vi "write_test_section_data.vi"(0 "dequeued data":T1={"Vapor Flow rate [g/s]"=0.0, "Liquid Flow rate [g/s]"=0.0, "Pressure/Temperature/Mixture Properties"={"Line Densities\n[g/cm^3]"={"Vapor Line"=0.15445189986836314, "Liquid Line"=0.25755261741892205}, "Mixture Properties"={"Enthalpy"=195841526251804.2, "Quality [-]"=-10.825375459319764}, "[Readings]"={"Streamwise P"=-3074.4228785963764, "Streamwise T"=nan, "Streamwise Sat P"=nan, "Streamwise Sat T"=nan, "Liquid Tank P"=3834985507386.06, "Liquid Tank T"=456.4106234658312, "Liquid Tank Sat P"=1736233577203.0627, "Liquid Tank Sat T"=492.17973224367375, "Separator P"=179910.46497250997, "Separator T"=-13120080.345725078, "Separator Sat P"=0.0, "Separator Sat T"=30.62899308837065, "Liquid Inlet P"=185261.09355383943, "Liquid Inlet T"=508.4593419640114, "Liquid Inlet Sat P"=12378986008470.418, "Liquid Inlet Sat T"=31.430570229281372, "Vapor Tank P"=108956.35947325415, "Vapor Tank T"=-10372083.904135285, "Vapor Tank Sat P"=0.0, "Vapor Tank Sat T"=16.912041354361705, "Vapor Inlet P"=379651.1166364239, "Vapor Inlet T"=381.53210552887515, "Vapor Inlet Sat P"=102884868683.01198, "Vapor Inlet Sat T"=51.054688909951395, "Upper Test Section P"=44976.833741485905, "Upper Test Section T"=-16719245.882515587, "Upper Test Section Sat P"=0.0, "Upper Test Section Sat T"=-7.288297090299707, "Lower Test Section P"=4027555317727.7935, "Lower Test Section T"=527.5685201983387, "Lower Test Section Sat P"=25461496462993.004, "Lower Test Section Sat T"=493.51977461723476}, "Condensor/Evaporator\nTemperature"={"Bottom Evaporator\nTemperature [C]"=0.011951520540655883, "Bottom Condensor\nTemperature [C]"=-36481825.305210106, "Top Evaporator\nTemperature [C]"=-0.005944396537208351, "Top Condensor\nTemperature [C]"=-0.03695927054192248}, "Test Section \nPressure [Pa]"=62496.106498599445, "Heater Temperatures [C]"={"Vapor Tank"=0.025136174921612436, "Liquid Tank"=0.021290742477967885}}, "Seconds Since \nSession Start"=0.0}, 1 "Loop Data Labels":string[](array[string])=["Vap Mass Flow", "Liq Mass Flow", "DP", "Liq Tank P", "LiqTank T", "Sep P", "SepT", "Liq In P", "Liq In T", "Vap Tank P", "Vap Tank T", "Dev Section P", "Dev Section T", "Up TS P", "Up TS T", "Low TS P", "Low TS T", "Cond Top T", "Evap Top T", "Cond Bot T", "Evap Bot T", "Win 3-4 P", "Top Heat T", "Bot Heat T"], 2 "Loop Data Index":dbl, 3 "Loop Data Prefix":string, 4 "Loop Data Folder":path) -> ()   [LabVIEW 2015]
uses:
  <vilib>/Utility/file.llb/Write Delimited Spreadsheet (DBL).vi
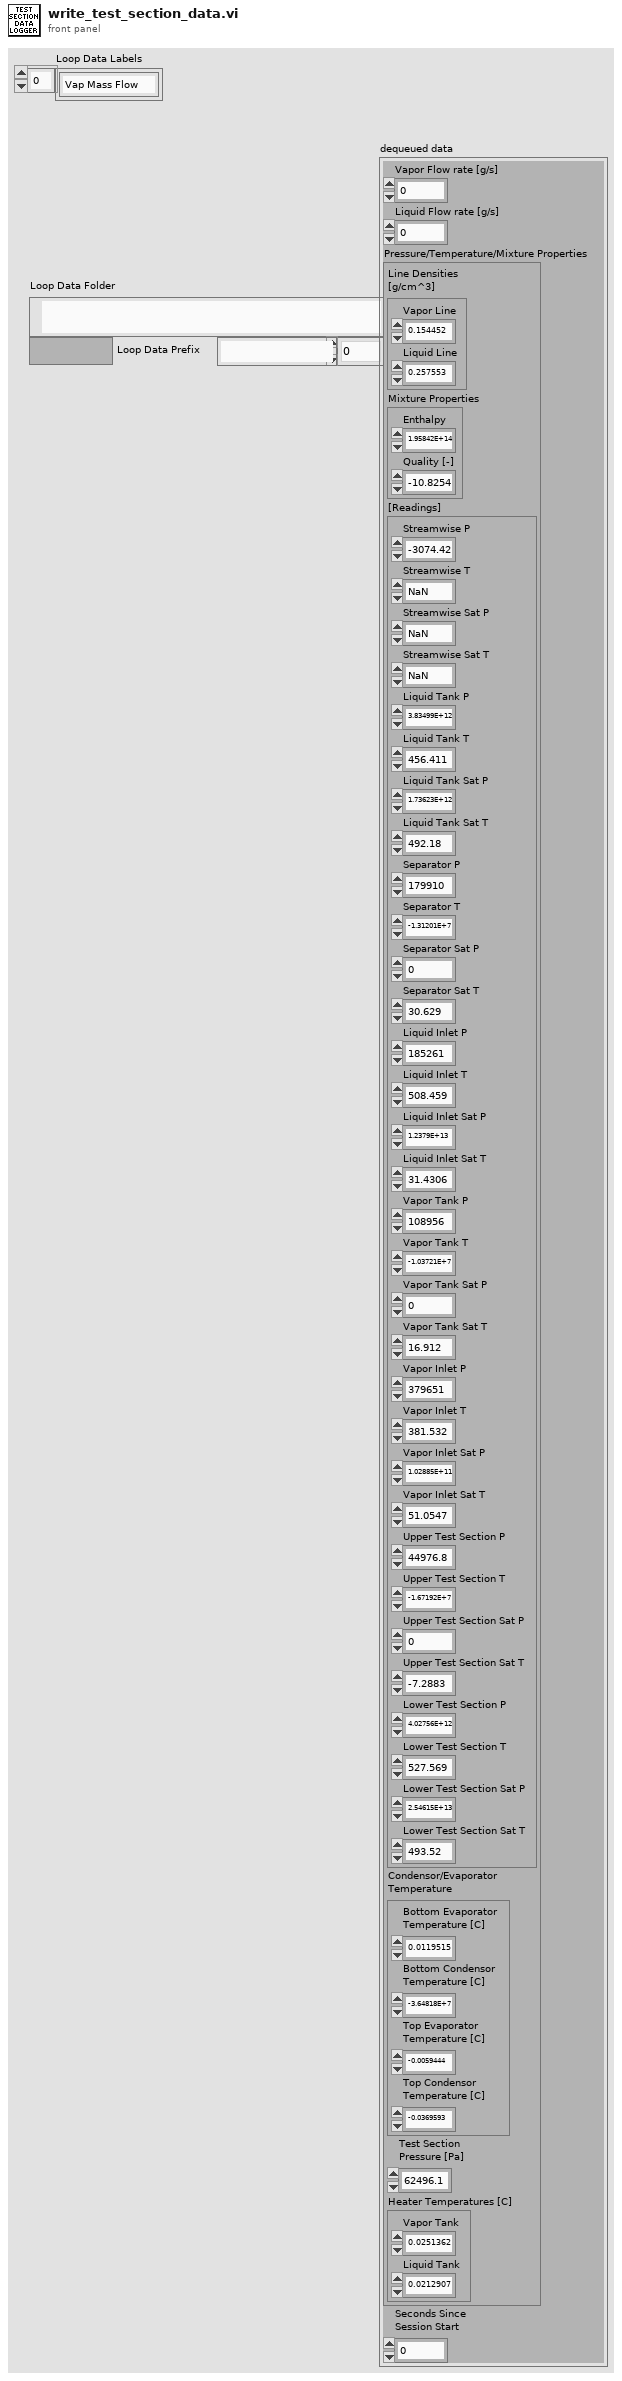
[diagram p1: front panel]
types:
  T1 = cluster{"Vapor Flow rate [g/s]":dbl, "Liquid Flow rate [g/s]":dbl, "Pressure/Temperature/Mixture Properties":cluster{"Line Densities\n[g/cm^3]":cluster{"Vapor Line":dbl, "Liquid Line":dbl}, "Mixture Properties":cluster{"Enthalpy":dbl, "Quality [-]":dbl}, "[Readings]":cluster{"Streamwise P":dbl, "Streamwise T":dbl, "Streamwise Sat P":dbl, "Streamwise Sat T":dbl, "Liquid Tank P":dbl, "Liquid Tank T":dbl, "Liquid Tank Sat P":dbl, "Liquid Tank Sat T":dbl, "Separator P":dbl, "Separator T":dbl, "Separator Sat P":dbl, "Separator Sat T":dbl, "Liquid Inlet P":dbl, "Liquid Inlet T":dbl, "Liquid Inlet Sat P":dbl, "Liquid Inlet Sat T":dbl, "Vapor Tank P":dbl, "Vapor Tank T":dbl, "Vapor Tank Sat P":dbl, "Vapor Tank Sat T":dbl, "Vapor Inlet P":dbl, "Vapor Inlet T":dbl, "Vapor Inlet Sat P":dbl, "Vapor Inlet Sat T":dbl, "Upper Test Section P":dbl, "Upper Test Section T":dbl, "Upper Test Section Sat P":dbl, "Upper Test Section Sat T":dbl, "Lower Test Section P":dbl, "Lower Test Section T":dbl, "Lower Test Section Sat P":dbl, "Lower Test Section Sat T":dbl}, "Condensor/Evaporator\nTemperature":cluster{"Bottom Evaporator\nTemperature [C]":dbl, "Bottom Condensor\nTemperature [C]":dbl, "Top Evaporator\nTemperature [C]":dbl, "Top Condensor\nTemperature [C]":dbl}, "Test Section \nPressure [Pa]":dbl, "Heater Temperatures [C]":cluster{"Vapor Tank":dbl, "Liquid Tank":dbl}}, "Seconds Since \nSession Start":dbl}
  T2 = cluster{"Line Densities\n[g/cm^3]":cluster{"Vapor Line":dbl, "Liquid Line":dbl}, "Mixture Properties":cluster{"Enthalpy":dbl, "Quality [-]":dbl}, "[Readings]":cluster{"Streamwise P":dbl, "Streamwise T":dbl, "Streamwise Sat P":dbl, "Streamwise Sat T":dbl, "Liquid Tank P":dbl, "Liquid Tank T":dbl, "Liquid Tank Sat P":dbl, "Liquid Tank Sat T":dbl, "Separator P":dbl, "Separator T":dbl, "Separator Sat P":dbl, "Separator Sat T":dbl, "Liquid Inlet P":dbl, "Liquid Inlet T":dbl, "Liquid Inlet Sat P":dbl, "Liquid Inlet Sat T":dbl, "Vapor Tank P":dbl, "Vapor Tank T":dbl, "Vapor Tank Sat P":dbl, "Vapor Tank Sat T":dbl, "Vapor Inlet P":dbl, "Vapor Inlet T":dbl, "Vapor Inlet Sat P":dbl, "Vapor Inlet Sat T":dbl, "Upper Test Section P":dbl, "Upper Test Section T":dbl, "Upper Test Section Sat P":dbl, "Upper Test Section Sat T":dbl, "Lower Test Section P":dbl, "Lower Test Section T":dbl, "Lower Test Section Sat P":dbl, "Lower Test Section Sat T":dbl}, "Condensor/Evaporator\nTemperature":cluster{"Bottom Evaporator\nTemperature [C]":dbl, "Bottom Condensor\nTemperature [C]":dbl, "Top Evaporator\nTemperature [C]":dbl, "Top Condensor\nTemperature [C]":dbl}, "Test Section \nPressure [Pa]":dbl, "Heater Temperatures [C]":cluster{"Vapor Tank":dbl, "Liquid Tank":dbl}}
  T3 = cluster{"Streamwise P":dbl, "Streamwise T":dbl, "Streamwise Sat P":dbl, "Streamwise Sat T":dbl, "Liquid Tank P":dbl, "Liquid Tank T":dbl, "Liquid Tank Sat P":dbl, "Liquid Tank Sat T":dbl, "Separator P":dbl, "Separator T":dbl, "Separator Sat P":dbl, "Separator Sat T":dbl, "Liquid Inlet P":dbl, "Liquid Inlet T":dbl, "Liquid Inlet Sat P":dbl, "Liquid Inlet Sat T":dbl, "Vapor Tank P":dbl, "Vapor Tank T":dbl, "Vapor Tank Sat P":dbl, "Vapor Tank Sat T":dbl, "Vapor Inlet P":dbl, "Vapor Inlet T":dbl, "Vapor Inlet Sat P":dbl, "Vapor Inlet Sat T":dbl, "Upper Test Section P":dbl, "Upper Test Section T":dbl, "Upper Test Section Sat P":dbl, "Upper Test Section Sat T":dbl, "Lower Test Section P":dbl, "Lower Test Section T":dbl, "Lower Test Section Sat P":dbl, "Lower Test Section Sat T":dbl}
  T4 = cluster{"Bottom Evaporator\nTemperature [C]":dbl, "Bottom Condensor\nTemperature [C]":dbl, "Top Evaporator\nTemperature [C]":dbl, "Top Condensor\nTemperature [C]":dbl}
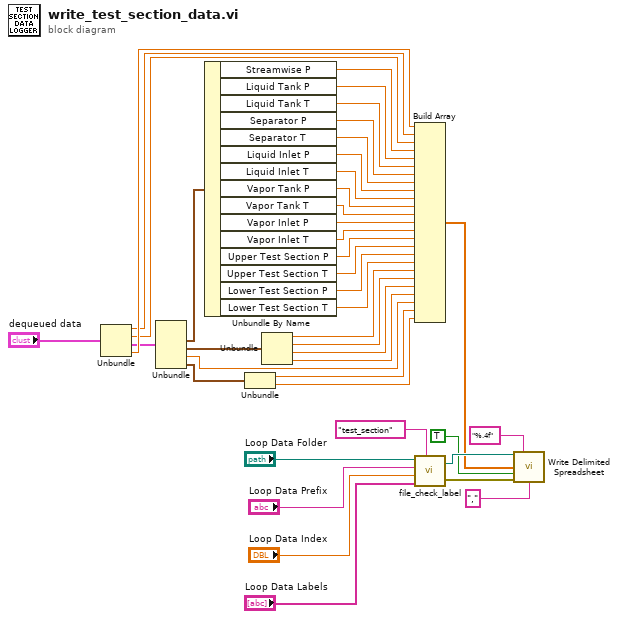
[diagram p0: block diagram]
diagram:
  n1 = Unbundle("dequeued data") -> ("Vapor Flow rate [g/s]"=w3:dbl, "Liquid Flow rate [g/s]"=w4:dbl, "Pressure/Temperature/Mixture Properties"=w5:T2, "Seconds Since \nSession Start"=w37:dbl)
  n2 = Unbundle(w5) -> ("[Readings]"=w6:T3, "Condensor/Evaporator\nTemperature"=w22:T4, "Test Section \nPressure [Pa]"=w27:dbl, "Heater Temperatures [C]"=w28:cluster{"Vapor Tank":dbl, "Liquid Tank":dbl})  [unwired: 2 out]
  n3 = Unbundle By Name(w6) -> ("Streamwise P"=w7:dbl, "Liquid Tank P"=w8:dbl, "Liquid Tank T"=w9:dbl, "Separator P"=w10:dbl, "Separator T"=w11:dbl, "Liquid Inlet P"=w12:dbl, "Liquid Inlet T"=w13:dbl, "Vapor Tank P"=w14:dbl, "Vapor Tank T"=w15:dbl, "Vapor Inlet P"=w16:dbl, "Vapor Inlet T"=w17:dbl, "Upper Test Section P"=w18:dbl, "Upper Test Section T"=w19:dbl, "Lower Test Section P"=w20:dbl, "Lower Test Section T"=w21:dbl)
  n4 = Unbundle(w28) -> ("Vapor Tank"=w29:dbl, "Liquid Tank"=w30:dbl)
  n5 = Unbundle(w22) -> ("Bottom Evaporator\nTemperature [C]"=w23:dbl, "Bottom Condensor\nTemperature [C]"=w24:dbl, "Top Evaporator\nTemperature [C]"=w25:dbl, "Top Condensor\nTemperature [C]"=w26:dbl)
  n6 = Build Array(w37, w3, w4, w7, w8, w9, w10, w11, w12, w13, w14, w15, w16, w17, w18, w19, w20, w21, w23, w24, w25, w26, w27, w29, w30) -> (w31:dbl[])
  n7 = call "file_check_label.vi"("base path"="Loop Data Folder", "prefix"="Loop Data Prefix", "index"="Loop Data Index", "Loop Data Labels"="Loop Data Labels", "task name"="test_section") -> ("dup path"=w35:path, "error out"=w36:errorcluster)
  n8 = call-poly <vilib>:"Write Delimited Spreadsheet.vi"("file path (dialog if empty)"=w35, "format (%.3f)"="%.4f", "1D data"=w31, "append to file? (new file:F)"=TRUE ("append to file? (F)"), "error in (no error)"=w36, "delimiter (\\t)"="," ("delimiter (\\t)")) -> ()  [unwired: 8 in, 2 out]
